vi "PmuAnalysis.vi"() -> ()   [LabVIEW 2018, in "Visualization.lvlib" / "VisualizeAnalysis.lvclass"]
uses:
  VisualizeAnalysis.lvclass
  <vilib>/event_ctls.llb/usereventprio.ctl
  VisualizeBase/VisualizeBase_class/Requests/VisUserEventType.ctl
  <extravilib>/ChannelInstances/Tag-bool/Write With Abort.vi
  <extravilib>/ChannelInstances/Tag-bool/Read With Abort.vi
  <extravilib>/ChannelInstances/Tag-bool/Instantiate.vi
  <vilib>/Utility/error.llb/Error Cluster From Error Code.vi
  <extravilib>/ChannelInstances/Tag-bool/Endpoint.vi
  <vilib>/Utility/file.llb/Read From Spreadsheet File (DBL).vi
  <extravilib>/ChannelInstances/Tag-bool/EndpointRead.vi
  <vilib>/ErrorRing/Error Ring.xnode
  <userlib>/NIST/NISTErrorLib/NISTErrorLib.lvlib
  VisualizeBase/VisualizeBase_class/VisualizeBase.lvclass
  Analysis/AnalysisModule/AnalysisModule.lvlib
  Visualization.lvlib
  Sensor/VisualizeSensor.lvclass
  <extravilib>/ChannelInstances/Tag-bool.lvlib
  TestClass/Test.lvclass
panel:
  in  "ModuleID":i32
  in  "btnClearTest":bool
  in  "btnReset":bool
  in  "btnPause":bool
  in  "btnOpen":bool
  in  "btnStop":bool
  in  "PluginName":string="Sensor.RoomAlert1"
  in  "Log Data":bool=TRUE
  out "Data from file":dbl[][](array[numeric])
  out "TVE":cluster{timestamp[], dbl[]}[](graph)
  out "FE":dbl(graph)=1.1347977483922023e-05
  out "ErrorArray":errorcluster[](array[cluster])
  out "RFE":dbl(graph)=-0.0019269131938461162
  out "Data real time":dbl[](array[numeric])
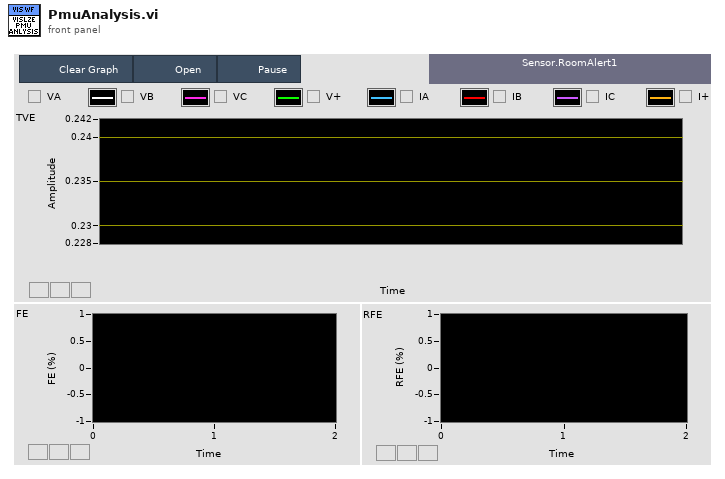
[diagram p1: front panel]
types:
  T1 = typedef "Visualization.lvlib/VisualizeBase.lvclass/VisRequestEvents.ctl" = cluster{"StopRequest":refnum<user-event>, "ResetRequest":refnum<user-event>, "FP Pop In or Out":refnum<user-event>}
  T2 = typedef "AnalysisModule.lvlib/clBroadcastEvents.ctl" = cluster{"DidInit":refnum<user-event>, "StatusUpdate":refnum<user-event>, "ErrorReport":refnum<user-event>, "DidStop":refnum<user-event>, "PathToINI":refnum<user-event>, "Config":refnum<user-event>, "ResultReport":refnum<user-event>, "FunctionClass":refnum<user-event>, "State":refnum<user-event>, "FunctionParams":refnum<user-event>, "Duration":refnum<user-event>}
  T3 = enum16{"open", "open or create", "create or replace", "create", "open (read-only)"}
  T4 = typedef "Visualization.lvlib/VisualizeBase.lvclass/VisUserEventType.ctl" = cluster{"BusIndex":i8, "Data":variant}
  T5 = typedef "usereventprio.ctl" = enum32{"high priority", "normal priority"}
  T6 = typedef "Tag-bool.lvlib/))Channel.ctl" = refnum<queue>
  T7 = typedef "sizeaction.ctl" = enum32{"Minimized", "Maximized", "Resized"}
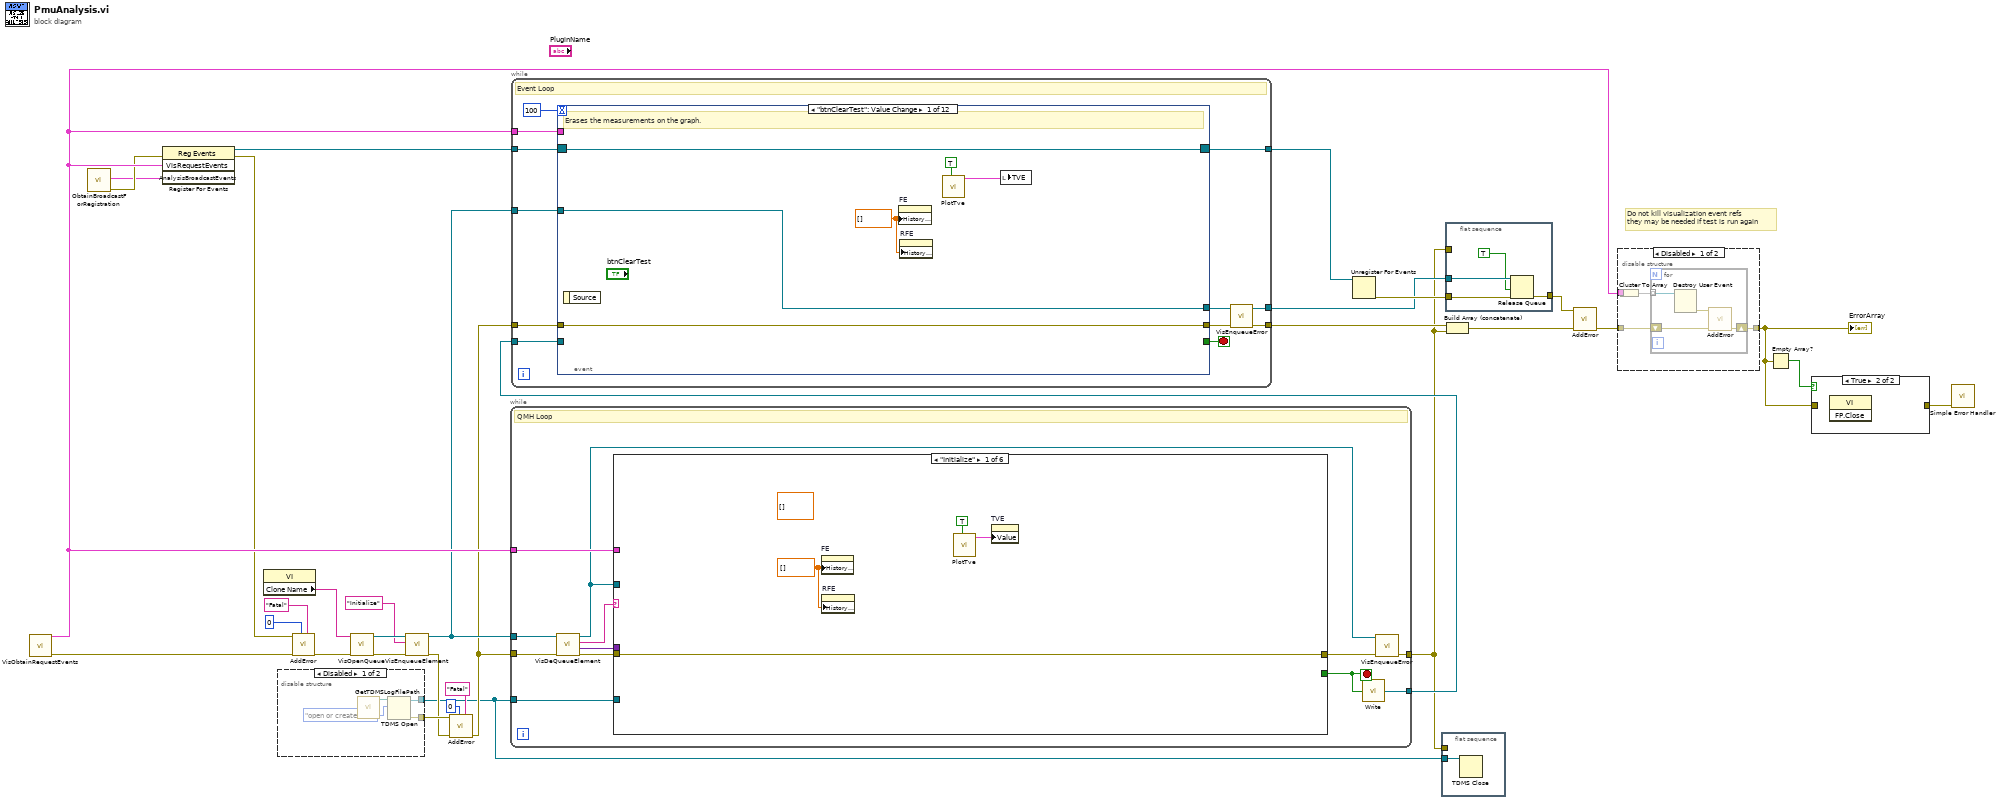
[diagram p0: block diagram]
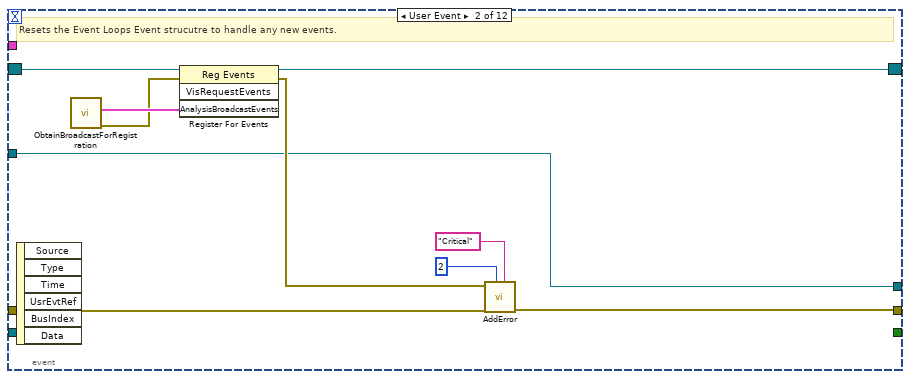
[diagram p4: hidden frame]
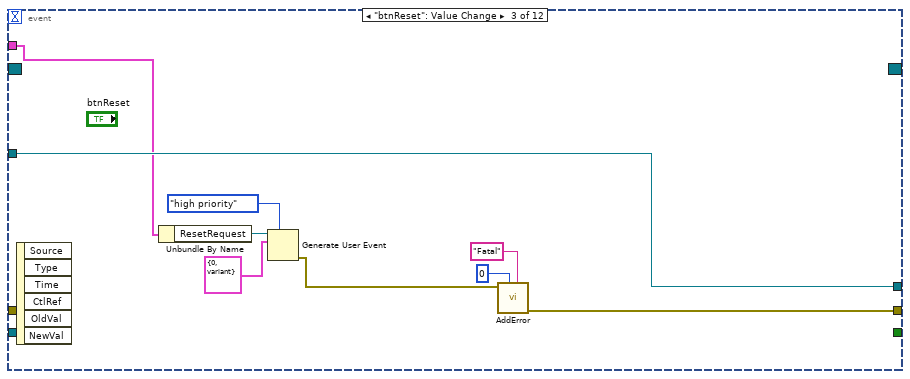
[diagram p5: hidden frame]
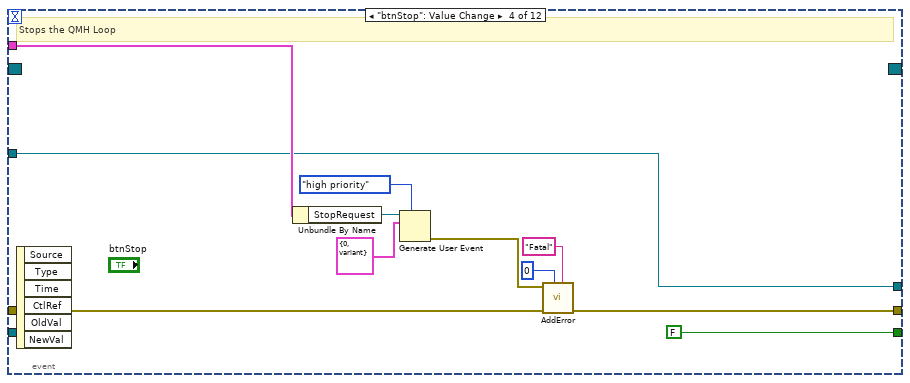
[diagram p6: hidden frame]
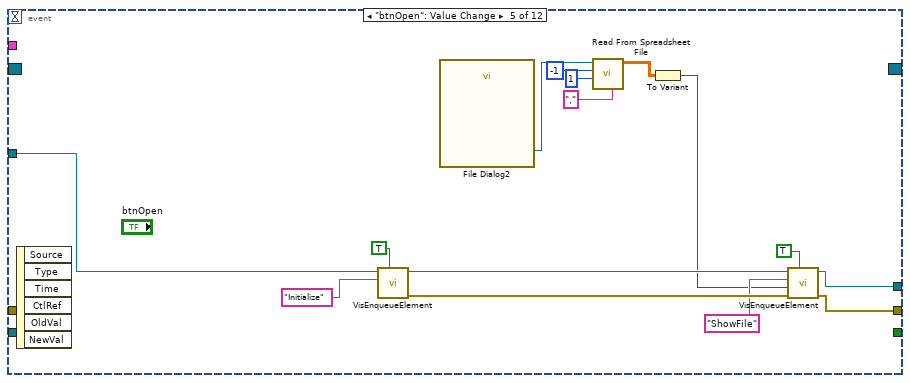
[diagram p7: hidden frame]
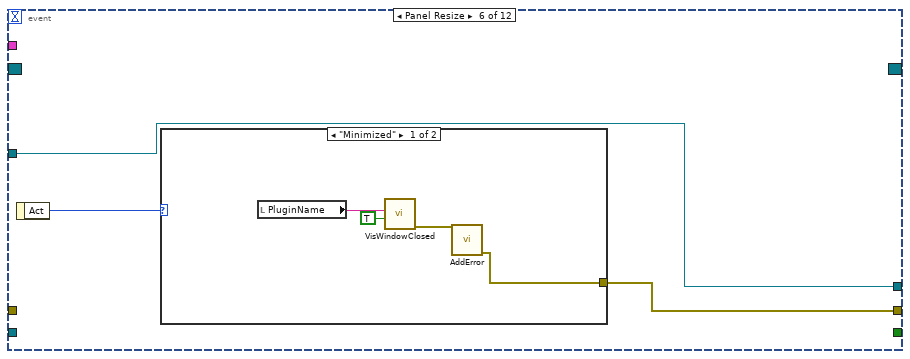
[diagram p8: hidden frame]
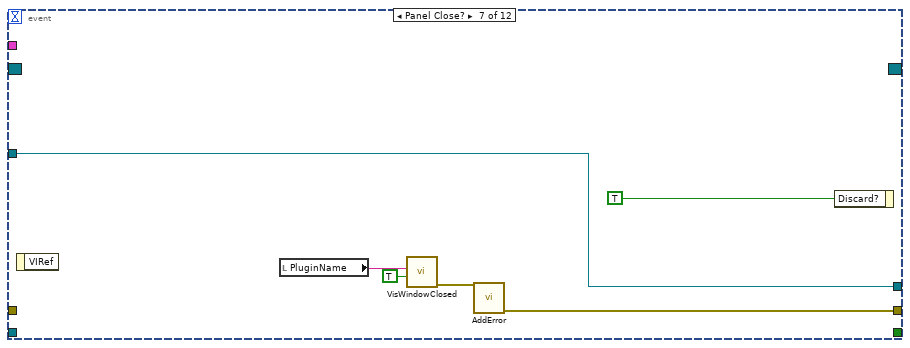
[diagram p10: hidden frame]
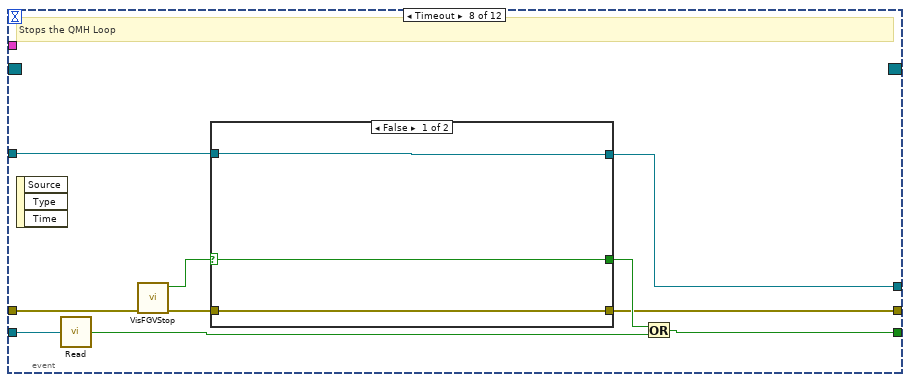
[diagram p11: hidden frame]
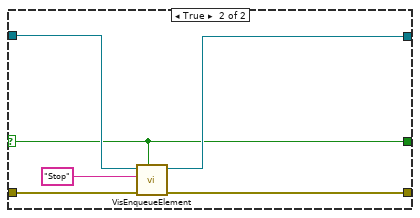
[diagram p12: hidden frame]
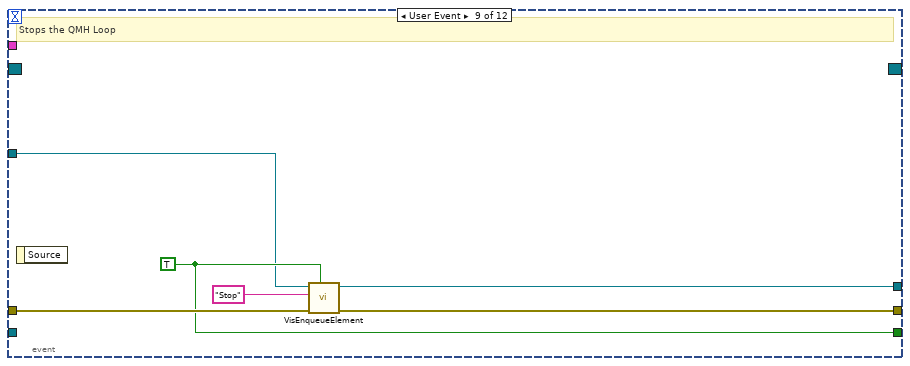
[diagram p13: hidden frame]
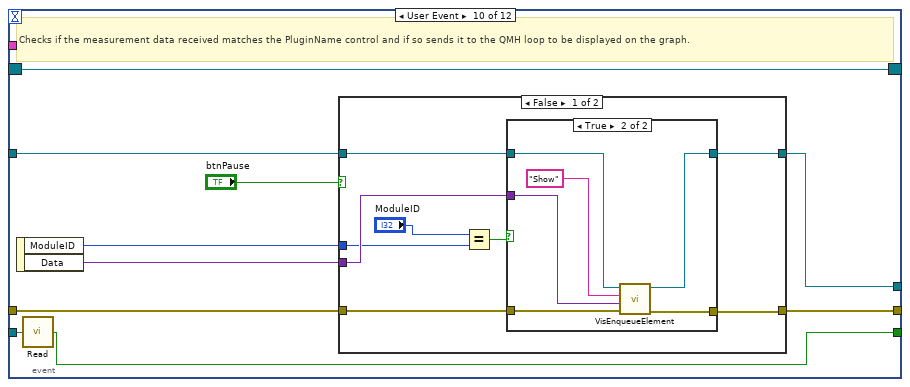
[diagram p14: hidden frame]
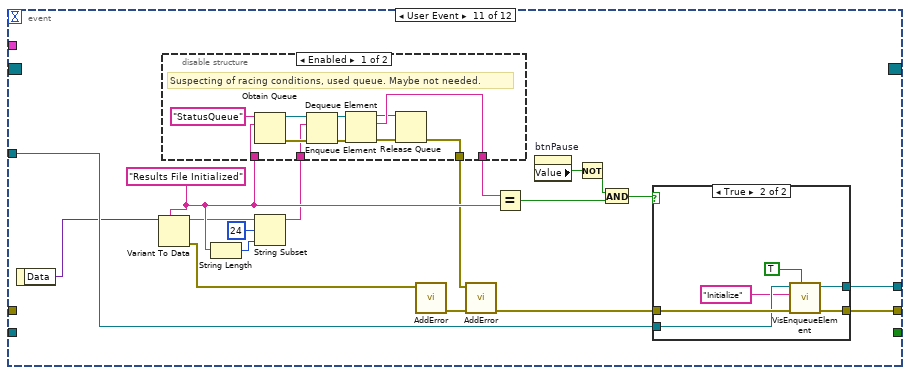
[diagram p17: hidden frame]
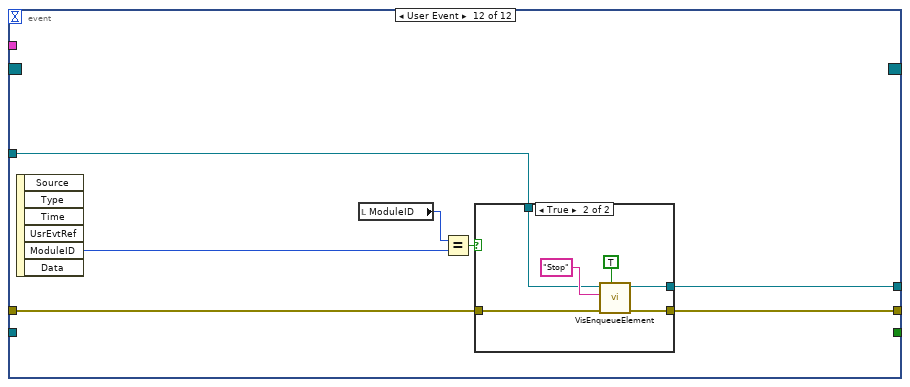
[diagram p20: hidden frame]
diagram:
  # "Do not kill visualization event refs\nthey may be needed if test is run again"
  n1 = call "VisObtainRequestEvents.vi"() -> ("Error"=w23:errorcluster[], "VisRequestEvents"=w25:T1)  [unwired: 10 in]
  n2 = call "ObtainBroadcastForRegistration.vi"() -> ("error out"=w3:errorcluster, "AnalysisBroadcastEvents"=w2:T2)  [unwired: 10 in]
  n3 = register-events(error in=w3, w25, w2) -> (reference out=w32:refnum<event-registration>, error out=w22:errorcluster)  [unwired: 1 in]
  n4 = property class="VI"() -> ("Clone Name"=w11:string)  [unwired: 2 in, 2 out]
  n5 = disable-structure shown="Disabled" {
    disable-tunnel: [w35 _] -> w8
    disable-tunnel: [w33 _] -> w5
    frame Disabled {
      n6 = call "GetTDMSLogFilePath.vi"() -> ("TDMS Log File Path"=w36:path)  [unwired: 11 in]
      n7 = TDMS Open(10:T3."open or create" ("operation (0:open)"), 11:w36) -> (0:w35:errorcluster, 3:w33:refnum<k34>)  [unwired: 5 in]
    }
    frame Enabled {
    }
  }
  n8 = call <userlib>:"AddError.vi"("Severity"="Fatal", "Priority"=u8 0, "ErrorArray In"=w23, "error in (no error)"=w22) -> ("ErrorArray Out"=w19:errorcluster[])  [unwired: 6 in, 1 out]
  n9 = call "VisOpenQueue.vi"("Error Array In"=w19, "QueueName"=w11) -> ("Error Array Out"=w17:errorcluster[], "queue out"=w18:refnum<queue>)  [unwired: 8 in]
  n10 = call "VisEnqueueElement.vi"("Error Array In"=w17, "Message"="Initialize", "queue in"=w18) -> ("Error Array Out"=w7:errorcluster[], "queue out"=w15:refnum<queue>)  [unwired: 7 in]
  n11 = call <userlib>:"AddError.vi"("Severity"="Fatal", "Priority"=u8 0, "ErrorArray In"=w7, "error in (no error)"=w8) -> ("ErrorArray Out"=w6:errorcluster[])  [unwired: 6 in, 1 out]
  n12 = while {
    tunnel: w6 -> [w42]
    tunnel: [w45] -> w4
    tunnel: w15 -> [w41]
    tunnel: w25 -> [w47]
    tunnel: [w38] -> w12
    tunnel: w5 -> [w37]
    stop <- w48 stop-if-true
    # "QMH Loop"
    n13 = call "VisDeQueueElement.vi"("Error Array In"=w42, "Queue In"=w41) -> ("Error Array Out"=w40:errorcluster[], "Data"=w43:variant, "Message"=w44:string, "Queue Out"=w39:refnum<queue>)  [unwired: 6 in]
    n14 = case shown="\"Initialize\"" w44 {
      selector: w44 -> [_ _ _ w106 _ _]
      tunnel: w43 -> [_ w55 w81 _ w125 _]
      tunnel: w40 -> [w52 w68 _ w104 _ w152]
      tunnel: [w52 w69 _ w103 w115 w152] -> w46
      tunnel: [_ _ _ _ w121 TRUE] -> w48
      tunnel: w47 -> [_ _ _ _ w120 _]
      tunnel: w39 -> [_ _ _ _ w119 _]
      tunnel: w37 -> [_ w63 _ _ _ _]
      frame "Initialize" {
        w51 = dbl[] [] ("History Data")
        (unwired) dbl[][] [] ("History Data")
        n15 = property on="FE" class="WFChart (strict)"("History Data"=w51) -> ()  [unwired: 2 in, 2 out]
        n16 = property on="RFE" class="WFChart (strict)"("History Data"=w51) -> ()  [unwired: 2 in, 2 out]
        n17 = call "PlotTve.vi"("Clear? (f)"=TRUE) -> ("TVE"=w49:cluster{timestamp[], dbl[]}[])  [unwired: 9 in, 1 out]
        n18 = property on="TVE" class="XYGraph (strict)"("Value"=w49) -> ()  [unwired: 2 in, 2 out]
      }
      frame "Show" {
        n19 = Variant To Data(type=dbl[] [], Variant=w55) -> (data=w60:dbl[], error out=w53:errorcluster)  [unwired: 1 in]
        "Data real time" <- w60
        n20 = call "PlotTve.vi"("error in (no error)"=w53, "Data real time"=w60) -> ("error out"=w54:errorcluster, "TVE"=→"TVE":cluster{timestamp[], dbl[]}[])  [unwired: 8 in]
        n21 = Index Array(array=w60, index #1=25 ("index"), index #2=26 ("index")) -> (element #1=→"FE":dbl, element #2=→"RFE":dbl)
        n22 = case shown="True" "Log Data" {
          tunnel: w54 -> [w70 w72]
          tunnel: [w70 w73] -> w65
          tunnel: w63 -> [_ w71]
          frame False {
          }
          frame True {
            # "Customize logging here for analysis"
            n23 = disable-structure shown="Disabled" {
              disable-tunnel: [w80 _] -> w73
              disable-tunnel: w72 -> [w79 _]
              disable-tunnel: w71 -> [w77 _]
              frame Disabled {
                n24 = call "PrepareWaveformDataForTDMS.vi"("error in (no error)"=w79) -> ("error out"=w76:errorcluster, "Measurement Data"=w74:dbl[][], "Channel Names"=w75:string[])  [unwired: 8 in]
                n25 = local read item#-1() -> (w78)
                n26 = TDMS Write(0:w77, 5:w78, 7:w75, 9:w74, 11:w76) -> (15:w80:errorcluster)  [unwired: 1 in, 3 out]
              }
              frame Enabled {
              }
            }
          }
        }
        n27 = call <userlib>:"AddError.vi"("Severity"="Fatal" ("String"), "Priority"=u8 0, "ErrorArray In"=w68, "error in (no error)"=w65) -> ("ErrorArray Out"=w69:errorcluster[])  [unwired: 6 in, 1 out]
      }
      frame "ShowFile" {
        n28 = Variant To Data(type=dbl[][] [], Variant=w81) -> (data=w94:dbl[][])  [unwired: 1 in, 1 out]
        "Data from file" <- w94
        n29 = Index Array(array=w94, index (col) #1=1 ("disabled index (col)"), index (col) #2=4 ("index (col)"), index (col) #3=7 ("index (col)"), index (col) #4=10 ("index (col)")) -> (element #1=w90:dbl[], element #2=w91:dbl[], element #3=w92:dbl[], element #4=w97:dbl[])  [unwired: 4 in]
        n30 = Index Array(array=w94, index (col) #1=25 ("disabled index (col)"), index (col) #2=26 ("index (col)")) -> (element #1=w95:dbl[], element #2=w96:dbl[])  [unwired: 2 in]
        n31 = Array Size(array=w97) -> (size(s)=w98:i32)
        n32 = Initialize Array(1.0 ("element"), w98) -> (w99:dbl[])
        n33 = property on="FE" class="WFChart (strict)"("History Data"=w95) -> ()  [unwired: 2 in, 2 out]
        n34 = Build Array(w90, w91, w92, w97, w99) -> (w93:dbl[][])
        n35 = property on="RFE" class="WFChart (strict)"("History Data"=w96) -> ()  [unwired: 2 in, 2 out]
        n36 = Transpose 2D Array(2D array=w93) -> ()  [unwired: 1 out]
      }
      frame Default {
        n37 = xnode "Error Ring"("parameter 0"=w106) -> ("error out"=w105:errorcluster)
        n38 = call <userlib>:"AddError.vi"("Severity"="Inform" ("String"), "Priority"=u8 5, "ErrorArray In"=w104, "error in (no error)"=w105) -> ("ErrorArray Out"=w103:errorcluster[], "error out"=w102:errorcluster)  [unwired: 6 in]
        n39 = call <vilib>:"Clear Errors.vi"("error in (no error)"=w102) -> ()  [unwired: 5 in, 2 out]
      }
      frame "Error" {
        n40 = Variant To Data(type=errorcluster[] [], Variant=w125) -> (data=w123:errorcluster[], error out=w114:errorcluster)  [unwired: 1 in]
        n41 = call <userlib>:"ParseErrors.vi"("ErrorArray"=w123) -> ("ErrorArray"=w122:errorcluster[])  [unwired: 8 in, 2 out]
        n42 = for {
          tunnel: w122 -> [w136] mode=indexing
          tunnel: [w130] -> w116 mode=concatenating
          tunnel: [w128] -> w121
          tunnel: w120 -> [w127]
          tunnel: w119 -> [w126]
          stop <- w128 stop-if-true
          n43 = call <userlib>:"GeneralHandler.vi"("error in (no error)"=w136) -> ("Severity"=w129:string, "Stop"=w133:bool, "Abort"=w134:bool, "Continue"=w135:bool)  [unwired: 6 in, 1 out]
          n44 = Build Array(w135, w134, w133) -> (w132:bool[])
          n45 = Boolean Array To Number(Boolean array=w132) -> (number=w131:u32)
          n46 = case shown="4" w131 {
            tunnel: [_ _ w141 w150] -> w130
            tunnel: w129 -> [_ _ _ w143]
            tunnel: [_ _ _ w145] -> w128
            tunnel: w127 -> [_ _ _ w144]
            tunnel: w126 -> [_ _ w137 _]
            frame 0, Default {
              # "No Dialog"
            }
            frame 1 {
              # "Continue"
            }
            frame 2 {
              # "Abort, Flush Queue"
              n47 = Flush Queue(queue=w137) -> (error out=w140:errorcluster)  [unwired: 1 in, 2 out]
              n48 = call <userlib>:"AddError.vi"("Severity"="Critical" ("String"), "Priority"=u8 1, "error in (no error)"=w140) -> ("ErrorArray Out"=w141:errorcluster[])  [unwired: 7 in, 1 out]
            }
            frame 4 {
              # "Stop"
              n49 = Unbundle By Name(w144) -> ("StopRequest"=w151:refnum<user-event>)
              n50 = Equal?(x=w143, y="Fatal" ("x")) -> (x = y?=w145:bool)
              n51 = Generate User Event(priority (normal)=usereventprio."high priority", user event=w151, event data cluster=T4 {"BusIndex"=0, "Data"=variant} ("event data")) -> (error out=w149:errorcluster)  [unwired: 1 in, 1 out]
              n52 = call <userlib>:"AddError.vi"("error in (no error)"=w149) -> ("ErrorArray Out"=w150:errorcluster[], "error out"=w146:errorcluster)  [unwired: 9 in]
              n53 = call <vilib>:"Clear Errors.vi"("error in (no error)"=w146) -> ()  [unwired: 5 in, 2 out]
            }
          }
        }
        n54 = call <userlib>:"AddError.vi"("Severity"="Critical", "Priority"=u8 2, "ErrorArray In"=w116, "error in (no error)"=w114) -> ("ErrorArray Out"=w115:errorcluster[])  [unwired: 6 in, 1 out]
      }
      frame "Stop" {
      }
    }
    n55 = call <extravilib>:"Write.vi"("element"=w48) -> ("channel"=w38:T6)  [unwired: 1 out]
    n56 = call "VisEnqueueError.vi"("Error Array In"=w46, "Queue in"=w39) -> ("Error Array Out"=w45:errorcluster[])  [unwired: 8 in, 1 out]
  }
  n57 = while {
    tunnel: w32 -> [w165]
    tunnel: [w159] -> w30
    tunnel: [w163] -> w31
    tunnel: w25 -> [w162]
    tunnel: w6 -> [w161]
    tunnel: w15 -> [w160]
    tunnel: [w156] -> w14
    tunnel: w12 -> [w154]
    stop <- w164 stop-if-true
    # "Event Loop"
    n58 = event shown="[0] \"btnClearTest\": Value Change" {
      selector: w165 -> [w170 w181 _ _ _ _ _ _ _ w260 _ _]
      dyn-events: [w170 w180 _ _ _ _ _ _ _ w260 _ _] -> w163
      timeout: 100 -> [_ _ _ _ _ _ _ _ _ _ _ _]
      tunnel: [_ _ _ FALSE ("Priority? (F)") _ _ _ w230 w251 w257 _ _] -> w164
      tunnel: [w171 w178 w184 w194 w203 w218 w224 w232 w253 w262 w285 w325] -> w158
      tunnel: w162 -> [_ _ w182 w193 _ _ _ _ _ _ _ _]
      tunnel: w161 -> [w171 w179 _ w201 _ _ _ w235 w254 w263 _ w323]
      tunnel: w160 -> [w169 w174 w183 w191 w211 w217 w228 w234 w249 w264 w287 w324]
      tunnel: [w169 w174 w183 w191 w202 w217 w228 w233 w252 w261 w284 w326] -> w157
      tunnel: w154 -> [_ _ _ _ _ _ _ w239 _ w258 _ _]
      event "btnClearTest": Value Change {
        w168 = dbl[] [] ("History Data")
        # "Erases the measurements on the graph."
        n59 = event-data() -> ()  [unwired: 1 in, 1 out]
        n60 = property on="FE" class="WFChart (strict)"("History Data"=w168) -> ()  [unwired: 2 in, 2 out]
        n61 = property on="RFE" class="WFChart (strict)"("History Data"=w168) -> ()  [unwired: 2 in, 2 out]
        n62 = call "PlotTve.vi"("Clear? (f)"=TRUE) -> ("TVE"=w167:cluster{timestamp[], dbl[]}[])  [unwired: 9 in, 1 out]
        n63 = local write "TVE"(w167) -> ()
      }
      event User Event {
        # "Resets the Event Loops Event strucutre to handle any new events."
        n64 = event-data() -> ()  [unwired: 1 in, 6 out]
        n65 = call "ObtainBroadcastForRegistration.vi"() -> ("error out"=w172:errorcluster, "AnalysisBroadcastEvents"=w173:T2)  [unwired: 10 in]
        n66 = register-events(reference=w181, error in=w172, w173) -> (reference out=w180:refnum<event-registration>, error out=w175:errorcluster)  [unwired: 1 in]
        n67 = call <userlib>:"AddError.vi"("Severity"="Critical", "Priority"=u8 2, "ErrorArray In"=w179, "error in (no error)"=w175) -> ("ErrorArray Out"=w178:errorcluster[])  [unwired: 6 in, 1 out]
      }
      event "btnReset": Value Change {
        n68 = event-data() -> ()  [unwired: 1 in, 6 out]
        n69 = Unbundle By Name(w182) -> ("ResetRequest"=w190:refnum<user-event>)
        n70 = Generate User Event(priority (normal)=usereventprio."high priority", user event=w190, event data cluster=T4 {"BusIndex"=0, "Data"=variant} ("event data")) -> (error out=w187:errorcluster)  [unwired: 1 in, 1 out]
        n71 = call <userlib>:"AddError.vi"("Severity"="Fatal", "Priority"=u8 0, "error in (no error)"=w187) -> ("ErrorArray Out"=w184:errorcluster[])  [unwired: 7 in, 1 out]
      }
      event "btnStop": Value Change {
        # "Stops the QMH Loop"
        n72 = event-data() -> ()  [unwired: 1 in, 6 out]
        n73 = Unbundle By Name(w193) -> ("StopRequest"=w199:refnum<user-event>)
        n74 = Generate User Event(priority (normal)=usereventprio."high priority", user event=w199, event data cluster=T4 {"BusIndex"=0, "Data"=variant} ("event data")) -> (error out=w200:errorcluster)  [unwired: 1 in, 1 out]
        n75 = call <userlib>:"AddError.vi"("Severity"="Fatal" ("String"), "Priority"=u8 0, "ErrorArray In"=w201, "error in (no error)"=w200) -> ("ErrorArray Out"=w194:errorcluster[])  [unwired: 6 in, 1 out]
      }
      event "btnOpen": Value Change {
        n76 = event-data() -> ()  [unwired: 1 in, 6 out]
        n77 = call "VisEnqueueElement.vi"("Priority? (F)"=TRUE, "Message"="Initialize", "queue in"=w211) -> ("Error Array Out"=w207:errorcluster[], "queue out"=w205:refnum<queue>)  [unwired: 7 in]
        n78 = call "File Dialog2"() -> ("selected path"=w212:path)  [unwired: 12 in, 3 out]
        n79 = call-poly <vilib>:"Read From Spreadsheet File.vi"("delimiter (\\t)"="," ("delimiter (\\t)"), "start of read offset (chars.:0)"=1, "number of rows (all:-1)"=-1, "file path (dialog if empty)"=w212) -> ("all rows"=w214:dbl[][])  [unwired: 3 in, 4 out]
        n80 = To Variant(anything=w214) -> (Variant=w204:variant)
        n81 = call "VisEnqueueElement.vi"("Priority? (F)"=TRUE, "Error Array In"=w207, "Data"=w204, "Message"="ShowFile", "queue in"=w205) -> ("Error Array Out"=w203:errorcluster[], "queue out"=w202:refnum<queue>)  [unwired: 5 in]
      }
      event Panel Resize {
        n82 = event-data() -> ("Act"=w219:T7)  [unwired: 1 in]
        n83 = case shown="\"Minimized\"" w219 {
          tunnel: [w220 _] -> w218
          frame "Minimized" {
            n84 = local read "PluginName"() -> (w222:string)
            n85 = call "VisWindowClosed.vi"("Window Closed?"=TRUE ("Window Minimized or Clozed?"), "Module Name"=w222) -> ("error out"=w223:errorcluster)  [unwired: 9 in]
            n86 = call <userlib>:"AddError.vi"("error in (no error)"=w223) -> ("ErrorArray Out"=w220:errorcluster[])  [unwired: 9 in, 1 out]
          }
          frame "Maximized", Default {
          }
        }
      }
      event Panel Close? {
        n87 = event-data() -> ()  [unwired: 1 in, 1 out]
        n88 = local read "PluginName"() -> (w225:string)
        n89 = call "VisWindowClosed.vi"("Window Closed?"=TRUE ("Window Minimized or Clozed?"), "Module Name"=w225) -> ("error out"=w227:errorcluster)  [unwired: 9 in]
        n90 = call <userlib>:"AddError.vi"("error in (no error)"=w227) -> ("ErrorArray Out"=w224:errorcluster[])  [unwired: 9 in, 1 out]
        n91 = event-data("Discard?"=TRUE) -> ()  [unwired: 1 in, 1 out]
      }
      event Timeout {
        # "Stops the QMH Loop"
        n92 = event-data() -> ()  [unwired: 1 in, 3 out]
        n93 = call <extravilib>:"Read.vi"("channel"=w239) -> ("element"=w231:bool)  [unwired: 1 in, 1 out]
        n94 = call "VisFGVStop.vi"("Error In"=w235) -> ("Error Out"=w237:errorcluster[], "Value"=w238:bool)  [unwired: 9 in]
        n95 = case shown="False" w238 {
          selector: w238 -> [w240 w243]
          tunnel: [w242 w246] -> w232
          tunnel: w237 -> [w242 w247]
          tunnel: w234 -> [w241 w245]
          tunnel: [w241 w244] -> w233
          tunnel: [w240 w243] -> w236
          frame False {
          }
          frame True {
            n96 = call "VisEnqueueElement.vi"("Priority? (F)"=w243, "Error Array In"=w247, "Message"="Stop", "queue in"=w245) -> ("Error Array Out"=w246:errorcluster[], "queue out"=w244:refnum<queue>)  [unwired: 6 in]
          }
        }
        n97 = Or(x=w236, y=w231) -> (x .or. y?=w230:bool)
      }
      event User Event {
        w251 = TRUE ("Priority? (F)")
        # "Stops the QMH Loop"
        n98 = event-data() -> ()  [unwired: 1 in, 1 out]
        n99 = call "VisEnqueueElement.vi"("Priority? (F)"=w251, "Error Array In"=w254, "Message"="Stop", "queue in"=w249) -> ("Error Array Out"=w253:errorcluster[], "queue out"=w252:refnum<queue>)  [unwired: 6 in]
      }
      event User Event {
        # "Checks if the measurement data received matches the PluginName control and if so sends it to the QMH loop to be displayed on the graph."
        n100 = event-data() -> ("ModuleID"=w255:i32, "Data"=w259:variant)  [unwired: 1 in]
        n101 = call <extravilib>:"Read.vi"("channel"=w258) -> ("element"=w257:bool)  [unwired: 1 in, 1 out]
        n102 = case shown="False" "btnPause" {
          tunnel: w264 -> [w272 w282]
          tunnel: w263 -> [w271 w281]
          tunnel: [w265 w281] -> w262
          tunnel: [w270 w282] -> w261
          tunnel: w259 -> [w269 _]
          tunnel: w255 -> [w268 _]
          frame False {
            n103 = Equal?(x="ModuleID", y=w268) -> (x = y?=w267:bool)
            n104 = case shown="True" w267 {
              tunnel: [w273 w279] -> w265
              tunnel: w272 -> [w274 w278]
              tunnel: w271 -> [w273 w280]
              tunnel: [w274 w276] -> w270
              tunnel: w269 -> [_ w277]
              frame False {
              }
              frame True {
                n105 = call "VisEnqueueElement.vi"("Error Array In"=w280, "Data"=w277, "Message"="Show", "queue in"=w278) -> ("Error Array Out"=w279:errorcluster[], "queue out"=w276:refnum<queue>)  [unwired: 6 in]
              }
            }
          }
          frame True {
          }
        }
      }
      event User Event {
        w297 = "Results File Initialized" ("Status")
        n106 = event-data() -> ("Data"=w286:variant)  [unwired: 1 in]
        n107 = Variant To Data(type=w297, Variant=w286) -> (data=w289:string, error out=w292:errorcluster)  [unwired: 1 in]
        n108 = String Length(string=w297) -> (length=w296:i32)
        n109 = String Subset(string=w289, offset (0)=24, length (rest)=w296) -> (substring=w294:string)
        n110 = disable-structure shown="Enabled" {
          disable-tunnel: [w304 w312] -> w290
          disable-tunnel: [w301 _] -> w293
          disable-tunnel: w294 -> [w306 w312]
          disable-tunnel: w297 -> [w305 _]
          frame Enabled {
            # "Suspecting of racing conditions, used queue. Maybe not needed."
            n111 = Obtain Queue(name (unnamed)="StatusQueue", element data type=w305) -> (queue out=w310:refnum<queue>, error out=w308:errorcluster)  [unwired: 3 in, 1 out]
            n112 = Enqueue Element(queue=w310, element=w306, error in (no error)=w308) -> (queue out=w309:refnum<queue>, error out=w307:errorcluster)  [unwired: 1 in, 1 out]
            n113 = Dequeue Element(queue=w309, error in (no error)=w307) -> (queue out=w303:refnum<queue>, element=w304:string, error out=w302:errorcluster)  [unwired: 1 in, 1 out]
            n114 = Release Queue(queue=w303, error in (no error)=w302) -> (error out=w301:errorcluster)  [unwired: 1 in, 2 out]
          }
          frame Disabled {
          }
        }
        n115 = call <userlib>:"AddError.vi"("error in (no error)"=w292) -> ("ErrorArray Out"=w291:errorcluster[])  [unwired: 9 in, 1 out]
        n116 = call <userlib>:"AddError.vi"("ErrorArray In"=w291, "error in (no error)"=w293) -> ("ErrorArray Out"=w288:errorcluster[])  [unwired: 8 in, 1 out]
        n117 = Equal?(x=w290, y=w297) -> (x = y?=w298:bool)
        n118 = property on="btnPause" class="Bool (strict)"() -> ("Value"=w299:bool)  [unwired: 2 in, 2 out]
        n119 = Not(x=w299) -> (.not. x?=w300:bool)
        n120 = And(x=w300, y=w298) -> (x .and. y?=w283:bool)
        n121 = case shown="True" w283 {
          tunnel: [w314 w319] -> w285
          tunnel: w288 -> [w314 w320]
          tunnel: w287 -> [w313 w318]
          tunnel: [w313 w315] -> w284
          frame False {
          }
          frame True {
            n122 = call "VisEnqueueElement.vi"("Priority? (F)"=TRUE, "Error Array In"=w320, "Message"="Initialize", "queue in"=w318) -> ("Error Array Out"=w319:errorcluster[], "queue out"=w315:refnum<queue>)  [unwired: 6 in]
          }
        }
      }
      event User Event {
        n123 = event-data() -> ("ModuleID"=w321:i32)  [unwired: 1 in, 5 out]
        n124 = local read "ModuleID"() -> (w322:i32)
        n125 = Equal?(x=w322, y=w321) -> (x = y?=w327:bool)
        n126 = case shown="True" w327 {
          tunnel: [w328 w333] -> w325
          tunnel: [w329 w332] -> w326
          tunnel: w324 -> [w329 w331]
          tunnel: w323 -> [w328 w330]
          frame False {
          }
          frame True {
            n127 = call "VisEnqueueElement.vi"("Priority? (F)"=TRUE, "Error Array In"=w330, "Message"="Stop", "queue in"=w331) -> ("Error Array Out"=w333:errorcluster[], "queue out"=w332:refnum<queue>)  [unwired: 6 in]
          }
        }
      }
    }
    n128 = call "VisEnqueueError.vi"("Error Array In"=w158, "Queue in"=w157) -> ("Error Array Out"=w159:errorcluster[], "Queue out"=w156:refnum<queue>)  [unwired: 8 in]
  }
  n129 = Unregister For Events(event registration refnum=w31) -> (error out=w29:errorcluster)  [unwired: 1 in]
  n130 = flat-sequence {
    tunnel: w5 -> [w336]
    tunnel: w4 -> [_]
    frame #0 {
      n131 = TDMS Close(11:w336) -> ()  [unwired: 1 in, 2 out]
    }
  }
  n132 = flat-sequence {
    tunnel: w29 -> [w340]
    tunnel: [w339] -> w27
    tunnel: w14 -> [w338]
    tunnel: w4 -> [_]
    frame #0 {
      n133 = Release Queue(queue=w338, force destroy? (F)=TRUE, error in (no error)=w340) -> (error out=w339:errorcluster)  [unwired: 2 out]
    }
  }
  n134 = Build Array (concatenate)(w30, w4) -> (w28:errorcluster[])
  n135 = call <userlib>:"AddError.vi"("ErrorArray In"=w28, "error in (no error)"=w27) -> ("ErrorArray Out"=w26:errorcluster[])  [unwired: 8 in, 1 out]
  n136 = disable-structure shown="Disabled" {
    disable-tunnel: w26 -> [w343 w349]
    disable-tunnel: w25 -> [w342 _]
    disable-tunnel: [w341 w349] -> w1
    frame Disabled {
      n137 = Cluster To Array(cluster=w342) -> (array=w344:refnum<user-event>[])
      n138 = for {
        tunnel: w344 -> [w348] mode=indexing
        shift-right: [w347] -> w341
        shift-left: w343 -> [w346]
        n139 = Destroy User Event(user event=w348) -> (error out=w345:errorcluster)  [unwired: 1 in]
        n140 = call <userlib>:"AddError.vi"("ErrorArray In"=w346, "error in (no error)"=w345) -> ("ErrorArray Out"=w347:errorcluster[])  [unwired: 8 in, 1 out]
      }
    }
    frame Enabled {
    }
  }
  "ErrorArray" <- w1
  n141 = Empty Array?(array=w1) -> (empty?=w24:bool)
  n142 = case shown="True" w24 {
    tunnel: [w350 _] -> w13
    tunnel: w1 -> [w351 _]
    frame False {
      n143 = Merge Errors(w351) -> (w350:errorcluster)
    }
    frame True {
      n144 = invoke class="VI" method="FP.Close"() -> ()  [unwired: 3 in, 3 out]
    }
  }
  n145 = call <vilib>:"Simple Error Handler.vi"("error in (no error)"=w13) -> ()  [unwired: 4 in, 5 out]
